vi "Joypad Loop.vi"() -> ()   [LabVIEW 2011]
doc: "This vi connects to a Joystick via Microsoft's Human Interface Devices and passes the necessary controls to the \"Remote\" variables \nSee Block Diagram:\n1. Quarry about available joystick\n2. Search for the joystick with the specified device\n3. If no match is found, then pass an error, then try and initialize the device\n4. Use a timed wile loop to save recourse, just looping and poling the joystick data is capable of high loop speeds\n5. Get Joystick sensor data\n6. Set the Trigger enable condition and pass along the XY data\n7. Normalize the values and use a running average to smooth out the control\n8. Apply expo weight for less sensitive control and zero out dead stick offset \n9. Set XY data\n10. XY plot is data binding to network variable for the XY plot on HUD from the Remote tab\n11. Use a stop button titled \"stop?\" so that the LabVIEW script can stop the vi\n12. Close the Joystick connection\n-Ruffin White\n-Kyle Green"
uses:
  <vilib>/Platform/TimedLoop/XDataNode/timing_clust.ctl
  <vilib>/Platform/TimedLoop/XDataNode/nitl_modes.ctl
  <vilib>/Platform/TimedLoop/XDataNode/wakeup.ctl
  BotCommands.ctl
  <vilib>/Utility/inputDevices.llb/closeJoystick.vi
  <vilib>/Utility/inputDevices.llb/joystickAcquire.vi
  <vilib>/Platform/TimedLoop/XDataNode/XDataNode.xnode
  <vilib>/Platform/TimedLoop/XDataNode/XDNodeRunTimeDep.lvlib
  Husky/clearpath_interface.lvlib
panel:
  in  "Tabs":enum32{"Speed Data", "Device Names", "Errors"}(tab)
  out "Speed":dbl(knob) scale=-1.0..1.0
  out "Rotation":dbl(knob) scale=1.0..-1.0
  in  "stop":bool
  in  "Stop Motors?":bool
  out "Msgs (total)":u32
  out "x":dbl
  out "y":dbl
  out "Increase Speed":bool
  out "Decrease Speed":bool
  out "Scaling Speed":dbl
  in  "Device Name":string="Controller (XBOX 360 For Windows)" caption="Give the exact \"device name\" string of the joypad you would like to use."
  in  "Husky":refnum<visa-resource-name>="ASRL1::INSTR"
  in  "error IO":errorcluster
  out "error out":errorcluster
  out "Network Timeout?":bool=TRUE
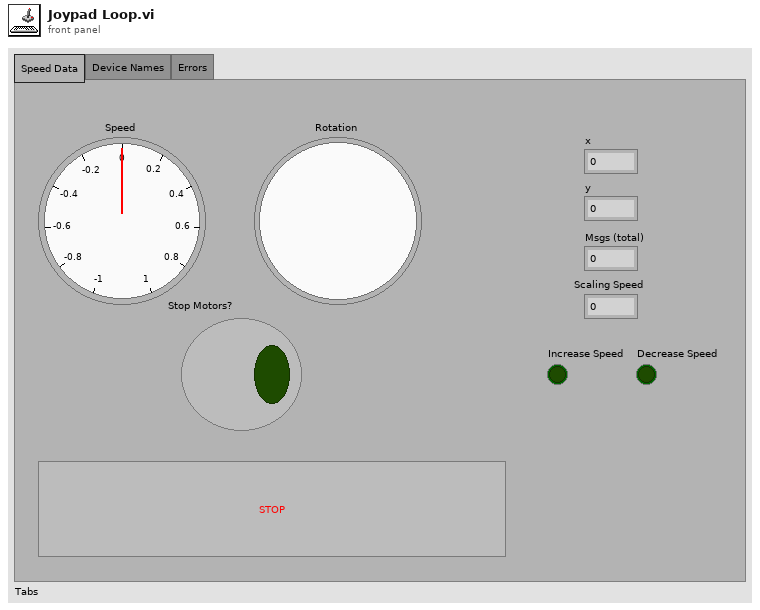
[diagram p1: front panel]
types:
  T1 = cluster{"axes total":u32, "buttons total":u32, "pov total":u32, "device name":string}[]
  T2 = cluster{"Xmit Queue":refnum<queue>, "Data Queue":refnum<queue>, "VISA resource name out":refnum<visa-resource-name>, "error out":errorcluster, "Message Data Cluster":cluster{"\nChar Idx":u8, "Num. Char Rem":u8, "Write Index":u8, "Read Index":u8, "Message Data Buffer":u8[][]}}
  T3 = typedef "XDNodeRunTimeDep.lvlib/timing_clust.ctl" = cluster{"Expected End [f-1]":u64, "Actual End [f-1]":u64, "Finished Late? [f-1]":bool, "Expected End [i-1]":u64, "Actual End [i-1]":u64, "Finished Late? [i-1]":bool, "Expected Start [i]":u64, "Actual Start [i]":u64, "Expected Start [f]":u64, "Actual Start [f]":u64, "Source Name":string, "Structure Name":string, "Period":i64, "Deadline":i64, "Offset":i64, "Start":i64, "Priority":i32, "Timeout":i32, "Mode":T4, "Wakeup Reason":T5, "Error":errorcluster, "Source Type":string, "Secondary Source Type":string, "Global End Time":u64, "Global Start Time":u64, "Frame Duration":u64, "Iteration Duration":u64, "Assigned CPU":i32, "I/O Scan Engine Mode":u32}
  T4 = typedef "XDNodeRunTimeDep.lvlib/nitl_modes.ctl" = enum32{"No Change", "Process missed periods, maintain original phase", "Discard missed periods, maintain original phase", "Process missed periods, ignore original phase", "Discard missed periods, ignore original phase"}
  T5 = typedef "XDNodeRunTimeDep.lvlib/wakeup.ctl" = enum32{"Normal", "Aborted", "Asynchronous wakeup", "Timing source error", "Timed loop error", "Timeout"}
  T6 = cluster{"X axis":i32, "Y axis":i32, "Z axis":i32, "X axis rotation":i32, "Y axis rotation":i32, "Z axis rotation":i32, "U axis":i32, "V axis":i32}
  T7 = cluster{"button 1":bool, "button 2":bool, "button 3":bool, "button 4":bool, "button 5":bool, "button 6":bool, "button 7":bool, "button 8":bool, "button 9":bool, "button 10":bool, "button 11":bool, "button 12":bool, "button 13":bool, "button 14":bool, "button 15":bool, "button 16":bool, "button 17":bool, "button 18":bool, "button 19":bool, "button 20":bool, "button 21":bool, "button 22":bool, "button 23":bool, "button 24":bool, "button 25":bool, "button 26":bool, "button 27":bool, "button 28":bool, "button 29":bool, "button 30":bool, "button 31":bool, "button 32":bool}
  T8 = typedef "BotCommands.ctl" = cluster{"Translational":dbl, "Rotational":dbl}
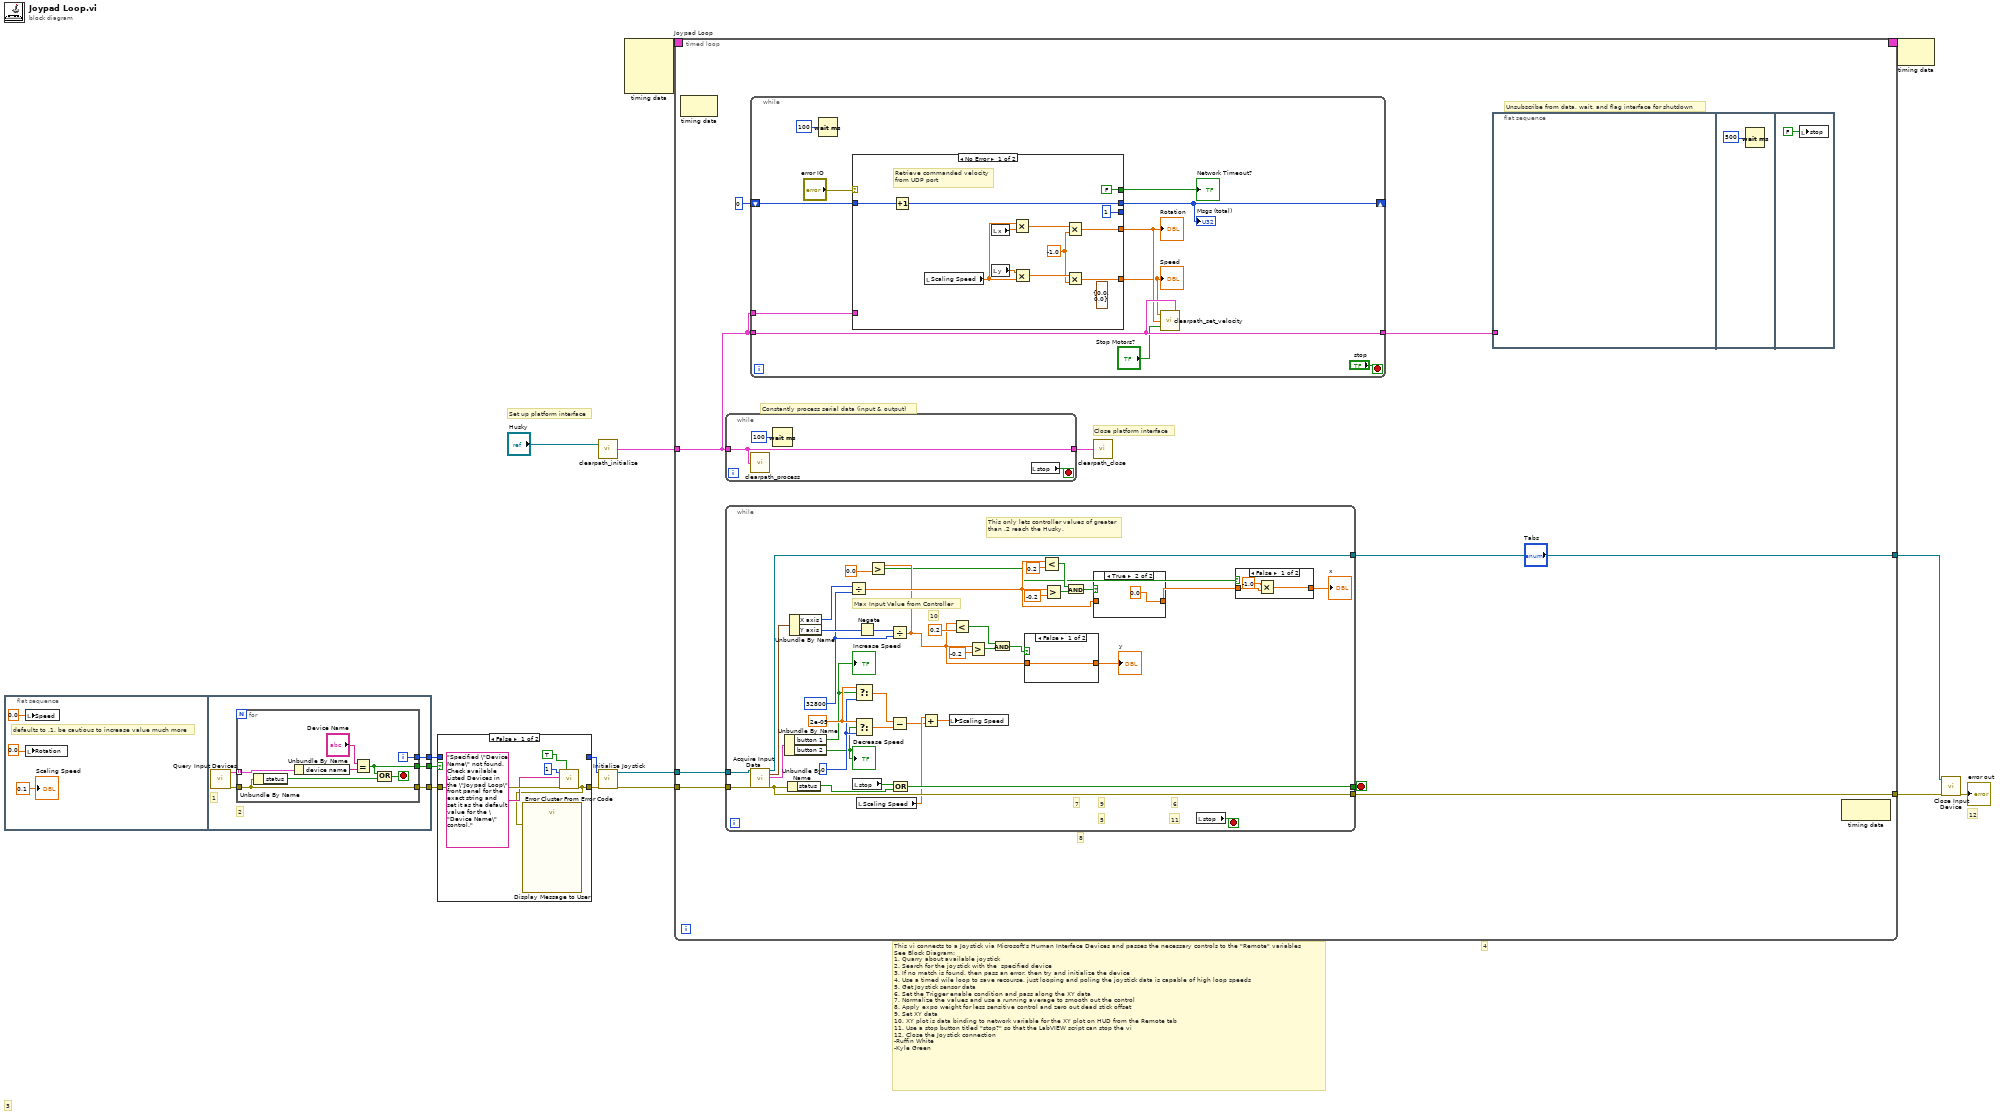
[diagram p0: block diagram]
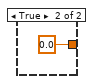
[diagram p3: hidden frame]
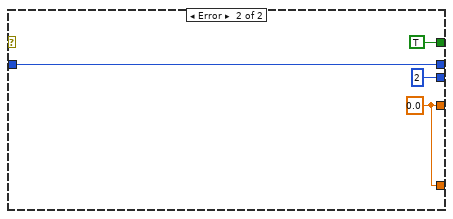
[diagram p5: hidden frame]
diagram:
  # "Set up platform interface"
  # "This vi connects to a Joystick via Microsoft's Human Interface Devices and passes the necessary controls to the \"Remote\" variables   \nSee Block Diagram:\n1.\tQuarry about available joystick\n2.\tSearch for the joystick with the  specified device\n3.\tIf no match is found, then pass an error, then try and initialize the device\n4.\tUse a timed wile loop to save recourse, just looping and poling the joystick data is capable of high loop speeds\n5.\tGet Joystick sensor data\n6.\tSet the Trigger enable condition and pass along the XY data\n7.\tNormalize the values and use a running average to smooth out the control\n8.\tApply expo weight for less sensitive control and zero out dead stick offset \n9.\tSet XY data\n10.\tXY plot is data binding to network variable for the XY plot on HUD from the Remote tab\n11.\tUse a stop button titled \"stop?\" so that the LabVIEW script can stop the vi\n12.\tClose the Joystick connection\n-Ruffin White\n-Kyle Green"
  # "12"
  # "4"
  # "3"
  n1 = flat-sequence {
    tunnel: [w21] -> w10
    tunnel: [w20] -> w9
    tunnel: [w18] -> w8
    frame #0 {
      # "defaults to .1. be cautious to increase value much more"
      n2 = local write "Speed"(0.0) -> ()
      n3 = local write "Rotation"(0.0) -> ()
      "Scaling Speed" <- 0.1
    }
    frame #1 {
      # "2"
      # "1"
      n4 = call <vilib>:"Query Input Devices.vi"() -> ("error out"=w19:errorcluster, "joystick info"=w22:T1)  [unwired: 8 in, 2 out]
      n5 = for {
        tunnel: w22 -> [w23] mode=indexing
        tunnel: [w28] -> w21
        tunnel: [w25] -> w20
        tunnel: w19 -> [w26]
        tunnel: [w26] -> w18
        i -> [w28]
        stop <- w27 stop-if-true
        n6 = Unbundle By Name(w26) -> ("status"=w24:bool)
        n7 = Unbundle By Name(w23) -> ("device name"=w29:string)
        n8 = Equal?(x="Device Name", y=w29) -> (x = y?=w25:bool)
        n9 = Compound Arithmetic op=OR(w25, w24) -> (w27:bool)
      }
    }
  }
  n10 = case shown="False" w9 {
    tunnel: w10 -> [_ w37]
    tunnel: [_ w37] -> w7
    tunnel: w8 -> [w35 w36]
    tunnel: [w31 w36] -> w3
    frame False {
      n11 = call <vilib>:"Error Cluster From Error Code.vi"("show call chain? (False)"=TRUE, "error in (no error)"=w35, "error message (\"\")"="Specified \"Device Name\" not found. Check available Listed Devices in the \"Joypad Loop\" front panel for the exact string and set it as the default value for the \"Device Name\" control." ("error message (\"\")"), "error code (0)"=1) -> ("error out"=w31:errorcluster)  [unwired: 5 in]
      n12 = call "Display Message to User"("error in (no error)"=w31) -> ()  [unwired: 9 in, 2 out]
    }
    frame True {
    }
  }
  n13 = call "clearpath_initialize.vi"("VISA resource name"="Husky") -> ("ClearpathComm"=w1:T2)  [unwired: 1 in]
  n14 = call <vilib>:"Initialize Joystick.vi"("error in (no error)"=w3, "device index"=w7) -> ("error out"=w11:errorcluster, "device ID"=w14:refnum<k1>)  [unwired: 8 in]
  n15 = node-c288() -> (w6:T3)  [unwired: 4 in]
  n16 = timed-loop "Joypad Loop" {
    tunnel: w14 -> [w46]
    tunnel: [w44] -> w12
    tunnel: w11 -> [w45]
    timing: w6 -> [_]
    timing-out: [_] -> w5
    tunnel: [w42] -> w4
    tunnel: w1 -> [w38]
    stop <- w43 stop-if-true
    # "Constantly process serial data (input & output)"
    # "Close platform interface"
    # "Unsubscribe from data, wait, and flag interface for shutdown"
    # "8"
    n17 = node-c288() -> ()  [unwired: 1 in, 1 out]
    n18 = while {
      tunnel: w38 -> [w97]
      tunnel: [w97] -> w39
      stop <- w95 stop-if-true
      n19 = call "clearpath_process.vi"("ClearpathComm"=w97) -> ()
      n20 = Wait (ms)(milliseconds to wait=u32 100) -> ()  [unwired: 1 out]
      n21 = local read "stop"() -> (w95:bool)
    }
    n22 = while {
      tunnel: w46 -> [w85]
      tunnel: w45 -> [w83]
      tunnel: [w82] -> w44
      tunnel: [w81] -> w43
      tunnel: [w79] -> w42
      stop <- w76 stop-if-true
      w55 = 32800
      w74 = 0
      w75 = 2e-05
      # "This only lets controller values of greater\nthan .2 reach the Husky."
      # "Max Input Value from Controller"
      # "7"
      # "11"
      # "10"
      # "9"
      # "6"
      # "5"
      n23 = call-poly <vilib>:"Acquire Input Data.vi"("device ID"=w85, "error in (no error)"=w83) -> ("device ID"=w79:refnum<k1>, "axis info"=w84:T6, "button info"=w86:T7, "error out"=w82:errorcluster)  [unwired: 13 in, 1 out]
      n24 = Unbundle By Name(w86) -> ("button 1"=w68:bool, "button 2"=w67:bool)
      "Increase Speed" <- w68
      "Decrease Speed" <- w67
      n25 = Unbundle By Name(w82) -> ("status"=w80:bool)
      n26 = Unbundle By Name(w84) -> ("X axis"=w53:i32, "Y axis"=w78:i32)
      n27 = Divide(x=w53, y=w55) -> (x/y=w52:dbl)
      n28 = local read "stop"() -> (w77:bool)
      n29 = Select(t=w75, s=w68, f=w74) -> (s? t:f=w73:dbl)
      n30 = Select(t=w75, s=w67, f=w74) -> (s? t:f=w72:dbl)
      n31 = local read "Scaling Speed"() -> (w71:dbl)
      n32 = Negate(x=w78) -> (-x=w54:i32)
      n33 = Divide(x=w54, y=w55) -> (x/y=w51:dbl)
      n34 = Greater?(x=w51, y=0.0) -> (0:w49:bool)
      n35 = Subtract(x=w73, y=w72) -> (x-y=w70:dbl)
      n36 = Compound Arithmetic op=OR(w77, w80) -> (w81:bool)
      n37 = Add(x=w71, y=w70) -> (x+y=w69:dbl)
      n38 = local write "Scaling Speed"(w69) -> ()
      n39 = Less?(x=w51, y=0.2) -> (x < y?=w58:bool)
      n40 = Greater?(x=w51, y=-0.2) -> (0:w57:bool)
      n41 = And(x=w58, y=w57) -> (x .and. y?=w56:bool)
      n42 = case shown="False" w56 {
        tunnel: [w91 0.0] -> w65
        tunnel: w51 -> [w91 _]
        frame False {
        }
        frame True {
        }
      }
      "y" <- w65
      n43 = Less?(x=w52, y=0.2) -> (x < y?=w63:bool)
      n44 = Greater?(x=w52, y=-0.2) -> (0:w62:bool)
      n45 = And(x=w63, y=w62) -> (x .and. y?=w61:bool)
      n46 = case shown="True" w61 {
        tunnel: w52 -> [w93 _]
        tunnel: [w93 0.0] -> w47
        frame False {
        }
        frame True {
        }
      }
      n47 = local read "stop"() -> (w76:bool)
      n48 = case shown="False" w49 {
        tunnel: [w87 w90] -> w48
        tunnel: w47 -> [w89 w90]
        frame False {
          n49 = Multiply(x=-1.0, y=w89) -> (x*y=w87:dbl)
        }
        frame True {
        }
      }
      "x" <- w48
    }
    n50 = while {
      tunnel: w38 -> [w106]
      tunnel: [w106] -> w41
      shift-right: [w103] -> _
      shift-left: 0 -> [w104]
      tunnel: w38 -> [w100]
      stop <- "stop" stop-if-true
      n51 = Wait (ms)(milliseconds to wait=u32 100) -> ()  [unwired: 1 out]
      n52 = case shown="No Error" "error IO" {
        tunnel: [w114 w124] -> w98
        tunnel: [w112 w124] -> w99
        tunnel: w100 -> [_ _]
        tunnel: [FALSE TRUE] -> w107
        tunnel: w104 -> [w119 w122]
        tunnel: [w118 w122] -> w103
        tunnel: [1 2] -> _
        frame No Error {
          w111 = -1.0
          (unwired) T8 {"Translational"=0.0, "Rotational"=0.0} ("BotCommands")
          # "Retrieve commanded velocity\nfrom UDP port"
          n53 = Increment(x=w119) -> (x+1=w118:i32)
          n54 = local read "Scaling Speed"() -> (w116:dbl)
          n55 = local read "x"() -> (w109:dbl)
          n56 = local read "y"() -> (w110:dbl)
          n57 = Multiply(x=w116, y=w109) -> (x*y=w113:dbl)
          n58 = Multiply(x=w110, y=w116) -> (x*y=w115:dbl)
          n59 = Multiply(x=w113, y=w111) -> (x*y=w112:dbl)
          n60 = Multiply(x=w115, y=w111) -> (x*y=w114:dbl)
        }
        frame Error {
          w124 = 0.0 ("Translational")
        }
      }
      "Speed" <- w98
      "Network Timeout?" <- w107
      "Msgs (total)" <- w103
      "Rotation" <- w99
      n61 = call "clearpath_set_velocity.vi"("ClearpathComm"=w106, "Zero Speeds"="Stop Motors?", "Rotational Speed"=w99, "Translational Speed"=w98) -> ()
    }
    n62 = call "clearpath_close.vi"("ClearpathComm"=w39) -> ()
    n63 = flat-sequence {
      tunnel: w41 -> [_]
      frame #0 {
      }
      frame #1 {
        n64 = Wait (ms)(milliseconds to wait=u32 500) -> ()  [unwired: 1 out]
      }
      frame #2 {
        n65 = local write "stop"(FALSE ("stop")) -> ()
      }
    }
    n66 = node-c288() -> ()  [unwired: 1 in, 1 out]
  }
  n67 = node-c288(w5) -> ()  [unwired: 1 out]
  n68 = call-poly <vilib>:"Close Input Device.vi"("error in (no error)"=w12, "device ID"=w4) -> ("error out"=→"error out":errorcluster)  [unwired: 8 in]
